vi "1.vi"() -> ()   [LabVIEW 2017]
panel:
  in  "stop":bool
  in  "open":bool
  out "text":string
  in  "file path (use dialog)":path
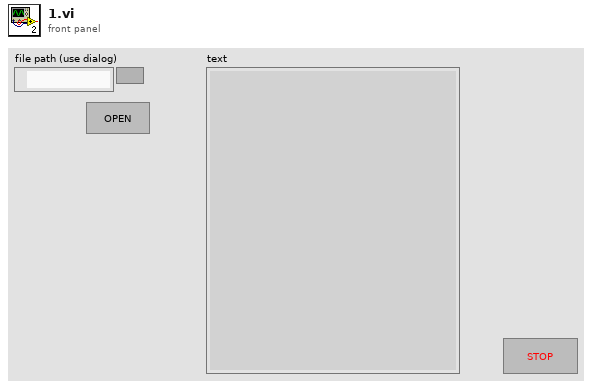
[diagram p1: front panel]
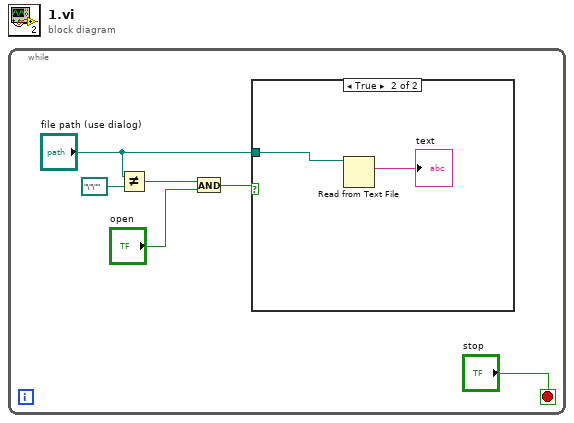
[diagram p0: block diagram]
diagram:
  n1 = while {
    stop <- "stop" stop-if-true
    n2 = Not Equal?(x="file path (use dialog)", y=path "\"\"") -> (x != y?=w5:bool)
    n3 = And(x=w5, y="open") -> (x .and. y?=w3:bool)
    n4 = case shown="True" w3 {
      tunnel: "file path (use dialog)" -> [_ w7]
      frame False {
      }
      frame True {
        n5 = Read from Text File(file (use dialog)=w7) -> (text=→"text":string)  [unwired: 3 in, 3 out]
      }
    }
  }
